vi "FuncImg-Initialise globals.vi"   [LabVIEW 2020]
uses:
  Typedefs/Get-Set-Clear Control.ctl
  Typedefs/Overlay FG functions.ctl
  ROI grouping window/Globals/gl_ROI grp window globals.vi
  Global variables/gl_Functional Imaging-Global variables.vi
types:
  T1 = typedef "Overlay FG functions.ctl" = enum16{"Generate new images", "Get stored images", "Clear"}
  T2 = typedef "Get-Set-Clear Control.ctl" = enum16{"Get", "Set", "Clear"}
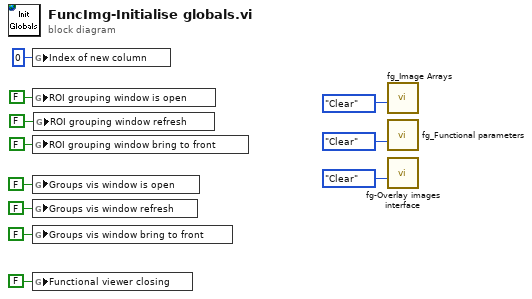
[diagram p0: block diagram]
diagram:
  n1 = global write "gl_ROI grp window globals.vi" "Index of new column"(0 ("Index of new column")) -> ()
  n2 = global write "gl_ROI grp window globals.vi" "ROI grouping window is open"(FALSE ("POI grouping window is open")) -> ()
  n3 = global write "gl_ROI grp window globals.vi" "ROI grouping window bring to front"(FALSE ("Bring POI grouping window to front")) -> ()
  n4 = global write "gl_ROI grp window globals.vi" "Groups vis window is open"(FALSE ("Groups vis window is open")) -> ()
  n5 = global write "gl_ROI grp window globals.vi" "Groups vis window refresh"(FALSE ("Groups vis window is open")) -> ()
  n6 = global write "gl_ROI grp window globals.vi" "Groups vis window bring to front"(FALSE ("Groups vis window bring to front")) -> ()
  n7 = global write "gl_Functional Imaging-Global variables.vi" "Functional viewer closing"(FALSE ("Functional viewer closing")) -> ()
  n8 = global write "gl_ROI grp window globals.vi" "ROI grouping window refresh"(FALSE ("POI grouping window is open")) -> ()
  n9 = call "fg_Image Arrays.vi"("Function"=Get-Set-Clear_Control."Clear") -> ()  [unwired: 9 in, 2 out]
  n10 = call "fg_Functional parameters.vi"("Function"=Get-Set-Clear_Control."Clear") -> ()  [unwired: 7 in, 4 out]
  n11 = call "fg-Overlay images interface.vi"("Function"=Overlay_FG_functions."Clear") -> ()  [unwired: 8 in, 3 out]
